vi "extract ROI CUDA.vi"(7 "ROI Descriptor":T2 {"Contours"."Type" items=["No Selection", "Point", "Line", "Rectangle", "Oval", "Polygon", "Freehand Region", "Annulus", "Unused2", "Unused3", "Broken Line", "Freehand Line", "Rotated Rectangle"]}, 10 "ROI":T1, 11 "CCD image ref":T1) -> (0 "yc":sgl, 1 "xc":sgl, 2 "img_out":sgl[][](array[numeric]), 4 "Y_base":sgl, 6 "X_base":sgl)   [LabVIEW 2017]
doc: "本VI的作用是将已有的ROI提取出图像，计算出图心，然后在图心上标记ROI的序号。\n本VI对ROI的实际尺寸不敏感，可以随意修改。\n本VI由于最终要出图给camera window，因此不建议并行多分支执行，最好是先执行完，后续提取出来的图再分成各个分支并行执行。"
uses:
  <vilib>/vision/Image Controls.llb/IMAQ Image.ctl
  <vilib>/vision/NI_Vision_Development_Module.lvlib
  <vilib>/Analysis/NI_AALBase.lvlib
  <vilib>/Analysis/Matrix/NI_Matrix.lvlib
  <vilib>/Analysis/baseanly.llb/Normalize Matrix.vi
  <vilib>/Analysis/Matrix/Numeric/Multiply/Multiply - RM,R.vi
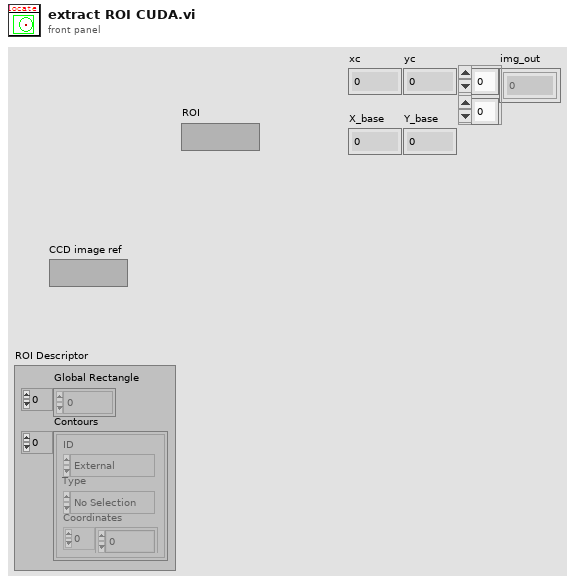
[diagram p1: front panel]
types:
  T1 = typedef "IMAQ Image.ctl" = refnum<image>
  T2 = typedef "ROI Descriptor" = cluster{"Global Rectangle":i32[], "Contours":cluster{"ID":enum32{"External", "Internal"}, "Type":u32, "Coordinates":i32[]}[]}
  T3 = typedef "IMAQ Rectangle" = cluster{"Left":i32, "Top":i32, "Right":i32, "Bottom":i32, "Rotation":dbl}
  T4 = typedef "NI_Matrix.lvlib/RealMatrix.ctl" = dbl[][]
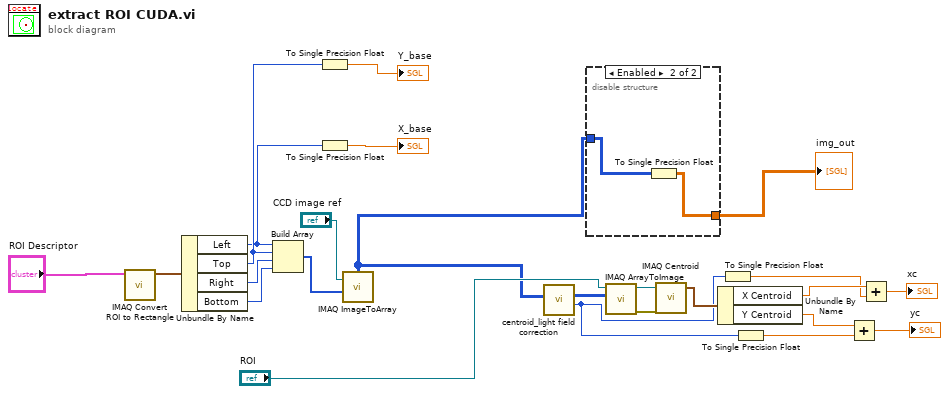
[diagram p0: block diagram]
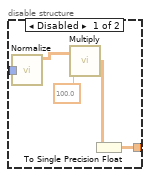
[diagram p2: hidden frame]
diagram:
  n1 = call "IMAQ Convert ROI to Rectangle"("ROI Descriptor"="ROI Descriptor") -> ("Rectangle"=w23:T3)  [unwired: 8 in, 1 out]
  n2 = Unbundle By Name(w23) -> ("Left"=w18:i32, "Top"=w20:i32, "Right"=w19:i32, "Bottom"=w22:i32)
  n3 = Build Array(w18, w20, w19, w22) -> (w21:i32[])
  n4 = To Single Precision Float(number=w20) -> (single precision float=→"Y_base":sgl)
  n5 = To Single Precision Float(number=w18) -> (single precision float=→"X_base":sgl)
  n6 = call "IMAQ ImageToArray"("Optional Rectangle"=w21, "Image"="CCD image ref") -> ("Image Pixels (U8)"=w1:u8[][])  [unwired: 2 in, 4 out]
  n7 = call "centroid_light field correction.vi"("ROI array (no trans)"=w1) -> ("xybase core"=w13:i32, "ROI array out"=w9:u8[][])  [unwired: 9 in]
  n8 = disable-structure shown="Enabled" {
    disable-tunnel: [w29 w30] -> w8
    disable-tunnel: w1 -> [w28 w31]
    frame Disabled {
      n9 = call-poly <vilib>:"Normalize.vi"("Matrix"=w28) -> ("Normalized Matrix"=w26:T4)  [unwired: 1 in, 3 out]
      n10 = call-poly <vilib>:"Multiply.vi"("Real Scalar c"=100.0 ("y"), "Real Matrix A"=w26) -> ("A * c"=w25:T4)
      n11 = To Single Precision Float(number=w25) -> (single precision float=w29:sgl[][])
    }
    frame Enabled {
      n12 = To Single Precision Float(number=w31) -> (single precision float=w30:sgl[][])
    }
  }
  "img_out" <- w8
  n13 = call "IMAQ ArrayToImage"("Image Pixels (U8)"=w9, "Image"="ROI") -> ("error out"=w10:errorcluster, "Image Out"=w3:T1)  [unwired: 8 in]
  n14 = call "IMAQ Centroid"("error in (no error)"=w10, "Image"=w3) -> ("Centroid"=w14:cluster{"X Centroid":sgl, "Y Centroid":sgl})  [unwired: 2 in, 1 out]
  n15 = Unbundle By Name(w14) -> ("X Centroid"=w11:sgl, "Y Centroid"=w12:sgl)
  n16 = To Single Precision Float(number=w13) -> (single precision float=w7:sgl)
  n17 = To Single Precision Float(number=w13) -> (single precision float=w6:sgl)
  n18 = Add(x=w12, y=w6) -> (x+y=→"yc":sgl)
  n19 = Add(x=w11, y=w7) -> (x+y=→"xc":sgl)
